vi "SLSCsortProperties.vi"(8 "Error In":errorcluster, 11 "properties":T1[](array[typedef])) -> (0 "Error Out":errorcluster, 1 "ReadWrite properties":T1[](array[typedef]), 2 "WriteOnly properties":T1[](array[typedef]), 3 "ReadOnly properties":T1[](array[typedef]))   [LabVIEW 2015]
doc: "This vi splits an array of SLSC properties into ReadOnly, WriteOnly and ReadWrite subarrays. Default if for access is ReadOnly.\nProperties of data type String will be filtered out."
uses:
  property.ctl
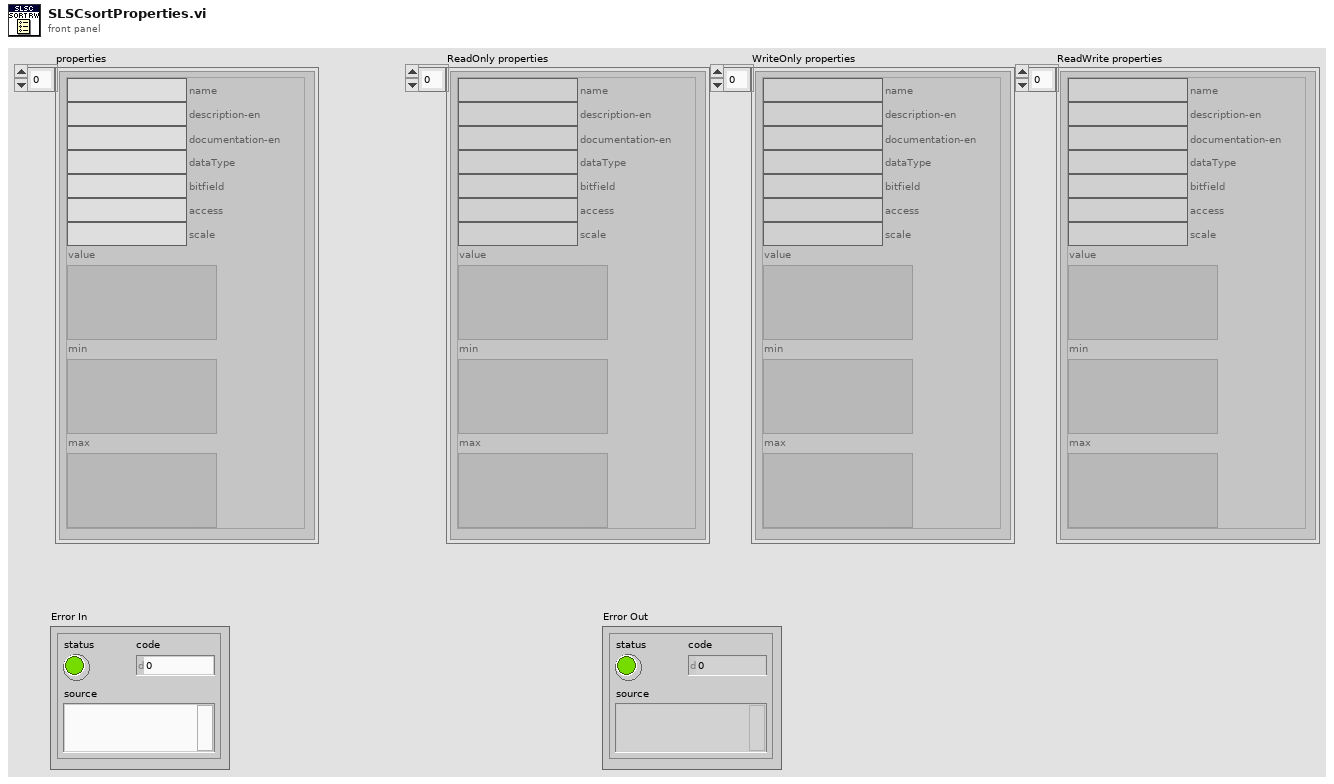
[diagram p1: front panel]
types:
  T1 = typedef "property.ctl" = cluster{"name":string, "description-en":string, "documentation-en":string, "dataType":string, "bitfield":string, "access":string, "scale":string, "value":variant, "min":variant, "max":variant}
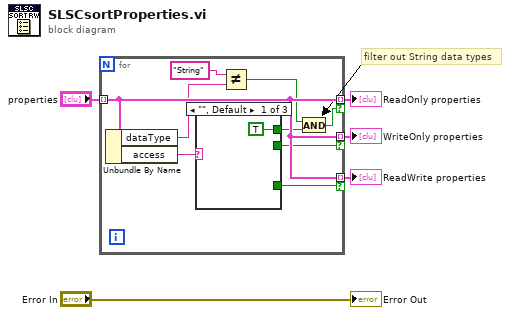
[diagram p0: block diagram]
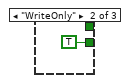
[diagram p2: hidden frame]
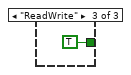
[diagram p3: hidden frame]
diagram:
  # "filter out String data types"
  n1 = for {
    tunnel: "properties" -> [w14] mode=indexing
    tunnel: [w14] -> w4 mode=indexing if=w7
    tunnel: [w14] -> w3 mode=indexing if=w12
    tunnel: [w14] -> w2 mode=indexing if=w11
    n2 = Unbundle By Name(w14) -> ("dataType"=w10:string, "access"=w13:string)
    n3 = case shown="\"\", Default" w13 {
      tunnel: [_ TRUE _] -> w12
      tunnel: [TRUE _ _] -> w8
      tunnel: [_ _ TRUE] -> w11
      frame "", Default {
      }
      frame "WriteOnly" {
      }
      frame "ReadWrite" {
      }
    }
    n4 = Not Equal?(x="String", y=w10) -> (x != y?=w6:bool)
    n5 = And(x=w6, y=w8) -> (x .and. y?=w7:bool)
  }
  "ReadOnly properties" <- w4
  "WriteOnly properties" <- w3
  "ReadWrite properties" <- w2
  "Error Out" <- "Error In"
